vi "tf FGV.vi"(10 "set tf":dbl, 11 "Enum":T1) -> (3 "tf":dbl)   [LabVIEW 2016, in "controllerLibrary.lvlib"]
uses:
  controllerLibrary.lvlib
  Controls/tf control.ctl
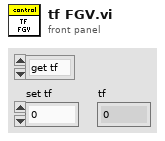
[diagram p1: front panel]
types:
  T1 = typedef "controllerLibrary.lvlib/tf control.ctl" = enum16{"get tf", "set tf"}
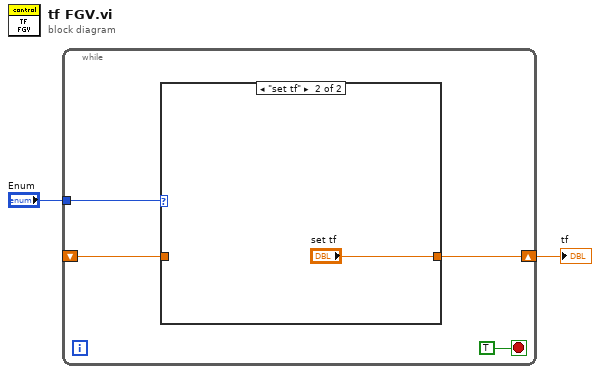
[diagram p0: block diagram]
diagram:
  n1 = while {
    tunnel: "Enum" -> [w5]
    shift-right: [w4] -> w2
    shift-left: _ -> [w3]
    stop <- TRUE stop-if-true
    n2 = case shown="\"set tf\"" w5 {
      tunnel: [w7 "set tf"] -> w4
      tunnel: w3 -> [w7 _]
      frame "get tf", Default {
      }
      frame "set tf" {
      }
    }
  }
  "tf" <- w2
